vi "Player Info.vi"(11 "Test in":refnum<class "Pattern 3.lvclass">) -> (0 "Defeat Speech":string, 1 "Victory Speech":string, 2 "Name":string, 3 "Test out":refnum<class "Pattern 3.lvclass">)   [LabVIEW 2015, in "Pattern 3.lvclass"]
uses:
  Pattern 3.lvclass
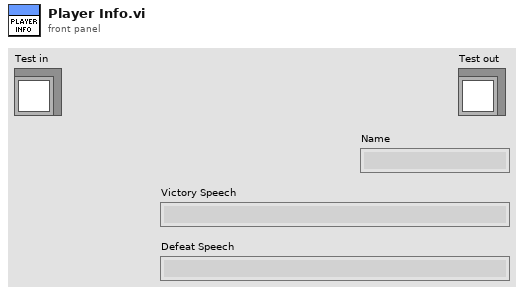
[diagram p1: front panel]
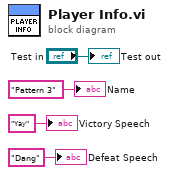
[diagram p0: block diagram]
diagram:
  "Test out" <- "Test in"
  "Name" <- "Pattern 3" ("Name")
  "Victory Speech" <- "Yay" ("Victory Speech")
  "Defeat Speech" <- "Dang" ("Defeat Speech")
